vi "Case.vi"(7 "ShiftR":refnum<class "ShiftR.lvclass">, 8 "error in":errorcluster, 9 "queue In":refnum<queue>, 11 "Close in":refnum<class "Close.lvclass">) -> (0 "error out":errorcluster, 1 "Exit":bool, 2 "Scrore":string, 3 "Close out":refnum<class "Close.lvclass">, 5 "ShiftR out":refnum<class "ShiftR.lvclass">)   [LabVIEW 2021, in "Msn Trasnsportation Library 1.lvlib" / "Close.lvclass"]
uses:
  Close.lvclass
  ShiftR/ShiftR.lvclass
  Abstract/Abstract.lvclass
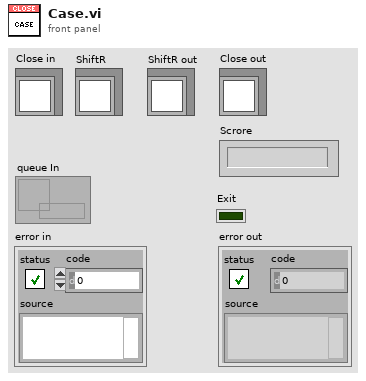
[diagram p1: front panel]
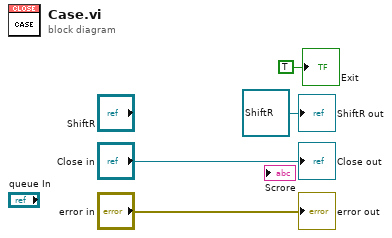
[diagram p0: block diagram]
diagram:
  "error out" <- "error in"
  "Close out" <- "Close in"
  "Exit" <- TRUE ("Exit")
  "ShiftR out" <- refnum<class "ShiftR.lvclass"> refnum ("ShiftR out")
